vi "BFS.vi"(7 "paths":i32[][][](array[numeric]), 11 "states":i32[][](array[numeric])) -> (1 "result path":i32[][](array[numeric]))   [LabVIEW 2021]
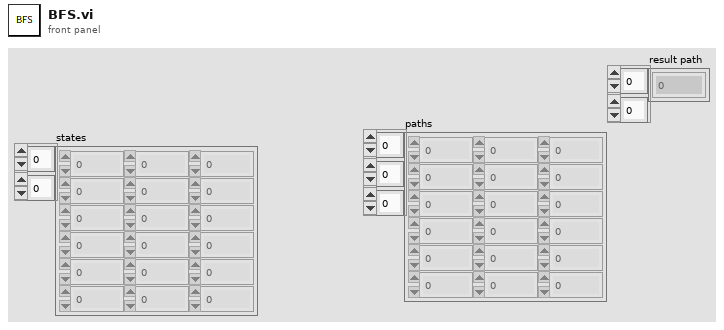
[diagram p1: front panel]
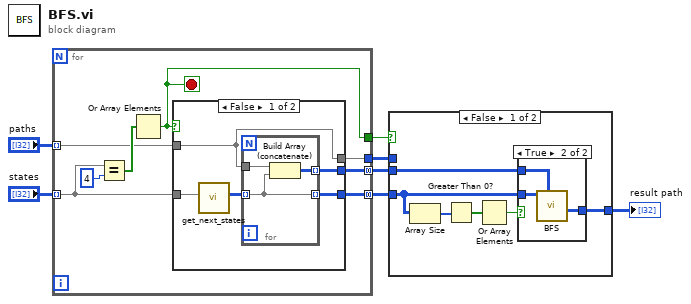
[diagram p0: block diagram]
diagram:
  n1 = for {
    tunnel: "states" -> [w13] mode=indexing
    tunnel: [w12] -> w6 mode=concatenating
    tunnel: [w11] -> w5
    tunnel: "paths" -> [w10] mode=indexing
    tunnel: [w9] -> w3 mode=concatenating
    tunnel: [w8] -> w2
    stop <- w11 stop-if-true
    n2 = Equal?(x=w13, y=4) -> (x = y?=w15:bool[])
    n3 = Or Array Elements(Boolean array=w15) -> (logical OR=w11:bool)
    n4 = case shown="False" w11 {
      tunnel: w13 -> [w20 _]
      tunnel: [w17 _] -> w12
      tunnel: w10 -> [w16 w24]
      tunnel: [w19 _] -> w9
      tunnel: [w16 w24] -> w8
      frame False {
        n5 = call "get_next_states.vi"("state"=w20) -> ("next states"=w18:i32[][])  [unwired: 10 in]
        n6 = for {
          tunnel: w16 -> [w23]
          tunnel: [w22] -> w19 mode=indexing
          tunnel: w18 -> [w21] mode=indexing
          tunnel: [w21] -> w17 mode=indexing
          n7 = Build Array (concatenate)(w23, w21) -> (w22:i32[][])
        }
      }
      frame True {
      }
    }
  }
  n8 = case shown="False" w5 {
    tunnel: w6 -> [w28 _]
    tunnel: w3 -> [w29 _]
    tunnel: w2 -> [_ w34]
    tunnel: [w30 w34] -> w1
    frame False {
      n9 = Array Size(array=w28) -> (size(s)=w27:i32[])
      n10 = Greater Than 0?(x=w27) -> (x > 0?=w26:bool[])
      n11 = Or Array Elements(Boolean array=w26) -> (logical OR=w25:bool)
      n12 = case shown="True" w25 {
        tunnel: [_ w33] -> w30
        tunnel: w29 -> [_ w32]
        tunnel: w28 -> [_ w31]
        frame False {
        }
        frame True {
          n13 = call "BFS.vi"("paths"=w32, "states"=w31) -> ("result path"=w33:i32[][])  [unwired: 9 in]
        }
      }
    }
    frame True {
    }
  }
  "result path" <- w1
